vi "Configure DC Resistance Range.vi"(8 "error in (no error)":errorcluster, 9 "DC Resistance Range (1: 100 Ohms)":i32(ring)=1 items=["10", "100", "1K", "10K", "100K"], 10 "Auto Range (T:Enable)":bool=TRUE, 11 "VISA resource name":refnum<visa-resource-name>) -> (0 "error out":errorcluster, 3 "VISA resource name out":refnum<visa-resource-name>)   [LabVIEW 2017, in "Agilent E4980.lvlib"]
doc: "Configures whether to enable the auto range function for DCR measurement, and selects the DCR range. \n\n<B>Notes:</B>\n(1) If you turn ON DC Bias when starting DCR measurement, DC Bias is automatically turned OFF. When the measurement parameter is Lp-Rdc or Ls-Rdc, you can not turn ON DC Bias. Otherwise, an error message appears."
uses:
  Agilent E4980.lvlib
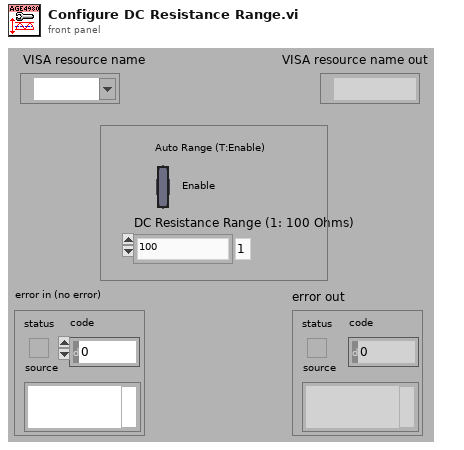
[diagram p1: front panel]
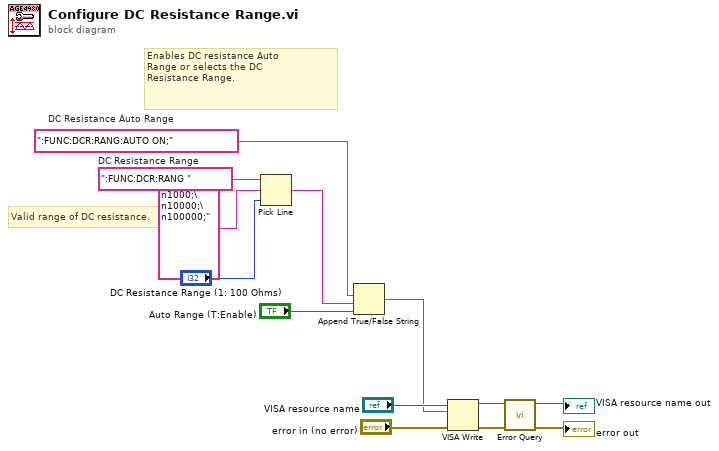
[diagram p0: block diagram]
diagram:
  w4 = ":FUNC:DCR:RANG "  # DC Resistance Range
  w12 = ":FUNC:DCR:RANG:AUTO ON;"  # DC Resistance Auto Range
  # "Enables DC resistance Auto\nRange or selects the DC\nResistance Range."
  # "Valid range of DC resistance."
  n1 = Pick Line(string ("")=w4, multi-line string="10;\n100;\n1000;\n10000;\n100000;", line index="DC Resistance Range (1: 100 Ohms)") -> (output string=w1:string)
  n2 = Append True/False String(1:"Auto Range (T:Enable)", 2:w1, 3:w12) -> (0:w7:string)  [unwired: 1 in]
  n3 = VISA Write(VISA resource name="VISA resource name", write buffer=w7, error in (no error)="error in (no error)") -> (VISA resource name out=w9:refnum<visa-resource-name>, error out=w8:errorcluster)  [unwired: 1 out]
  n4 = call "Error Query.vi"("error in (no error)"=w8, "VISA resource name"=w9) -> ("error out"=→"error out":errorcluster, "VISA resource name out"=→"VISA resource name out":refnum<visa-resource-name>)  [unwired: 6 in, 2 out]
